vi "Main.vi"() -> ()   [LabVIEW 2018]
uses:
  Source/SG/Typedefs/Waveform Timing Configuration.ctl
  Source/SG/Typedefs/Instrument Configuration.ctl
  <instrlib>/niRFSG/niRFSG.llb/niRFSG Ref Clock Sources.ctl
  <instrlib>/niRFSG/niRFSG.llb/niRFSG Trigger Terminals.ctl
  Source/SG/Typedefs/PAEN Configuration.ctl
  <instrlib>/niRFSG/niRFSG.llb/niRFSG Exported Signal Destinations.ctl
  <instrlib>/niDigital/niDigital.llb/niDigital Burst Pattern (Burst Only).vi
  Source/SG/SG.lvlib
  Source/Digital/Digital.lvlib
panel:
  in  "Configurations":enum32{"Hardware", "Waveform Generation"}(tab)=enum."Waveform Generation"
  in  "RFSG Resource":refnum<k15>="VST2"
  in  "NI Digital Resource":refnum<k15>="PXIe-6570"
  in  "Waveform Timing Configuration":T1={"Duty Cycle (%)"=99.0, "Pre-Burst Time (s)"=1e-06, "Post-Burst Time (s)"=1e-06} {"Post-Burst Time (s)" format="%#_6p"; "Pre-Burst Time (s)" format="%#_6p"; "Duty Cycle (%)" min=1.0 max=100.0 step=1.0 format="%#_2d%%"}
  in  "Waveform File Path":path
  in  "External Attenuation (dB)":dbl
  in  "DUT Average Input Power (dBm)":dbl=-20.0
  in  "Carrier Frequency (Hz)":dbl=1000000000.0 format="%#_6p"
  in  "stop":bool
  out "Status":string
  # "Only supports NI-5840 for generation"
  # "Will use local file if empty"
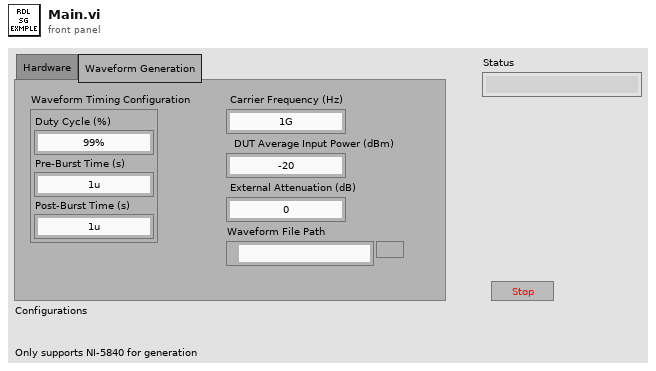
[diagram p1: front panel]
types:
  T1 = typedef "SG.lvlib/Waveform Timing Configuration.ctl" = cluster{"Duty Cycle (%)":dbl, "Pre-Burst Time (s)":dbl, "Post-Burst Time (s)":dbl}
  T2 = typedef "SG.lvlib/Instrument Configuration.ctl" = cluster{"Reference Clock Source":T3, "Carrier Frequency (Hz)":dbl, "DUT Average Input Power (dBm)":dbl, "External Attenuation (dB)":dbl, "Marker 0 Export Terminal":T4, "Share LO  SG->SA":bool}
  T3 = typedef "niRFSG Ref Clock Sources.ctl" = string
  T4 = typedef "niRFSG Trigger Terminals.ctl" = string
  T5 = typedef "SG.lvlib/PAEN Configuration.ctl" = cluster{"PAEN Mode":enum16{"Disabled", "Static", "Dynamic"}, "Command Enable Time (s)":dbl, "Command Disable Time (s)":dbl, "PA Enable Trigger Mode":i32, "PA Enable Trigger Export Terminal":T6}
  T6 = typedef "niRFSG Exported Signal Destinations.ctl" = string
  T7 = cluster{"Generation":cluster{"SG Configuration":T2, "Timing Configuration":T1, "PAEN Configuration":T5}, "Example Folder Path":path}
  T8 = typedef "SG.lvlib/Waveform.ctl" = cluster{"Waveform Name":string, "Waveform":cluster{"x0":dbl, "dx":dbl, "y":csg[]}, "Signal Bandwidth (Hz)":dbl, "PAPR (dB)":dbl, "Burst Length (s)":dbl, "Sample Rate":dbl, "Burst Start Locations":i32[], "Burst Stop Locations":i32[], "Idle Duration Present?":bool}
  T9 = typedef "Digital.lvlib/Project Files.ctl" = cluster{"Pin Map File":path, "Specifications Files":path[], "Pin Levels Files":path[], "Timing Files":path[], "Digital Pattern Files":path[]}
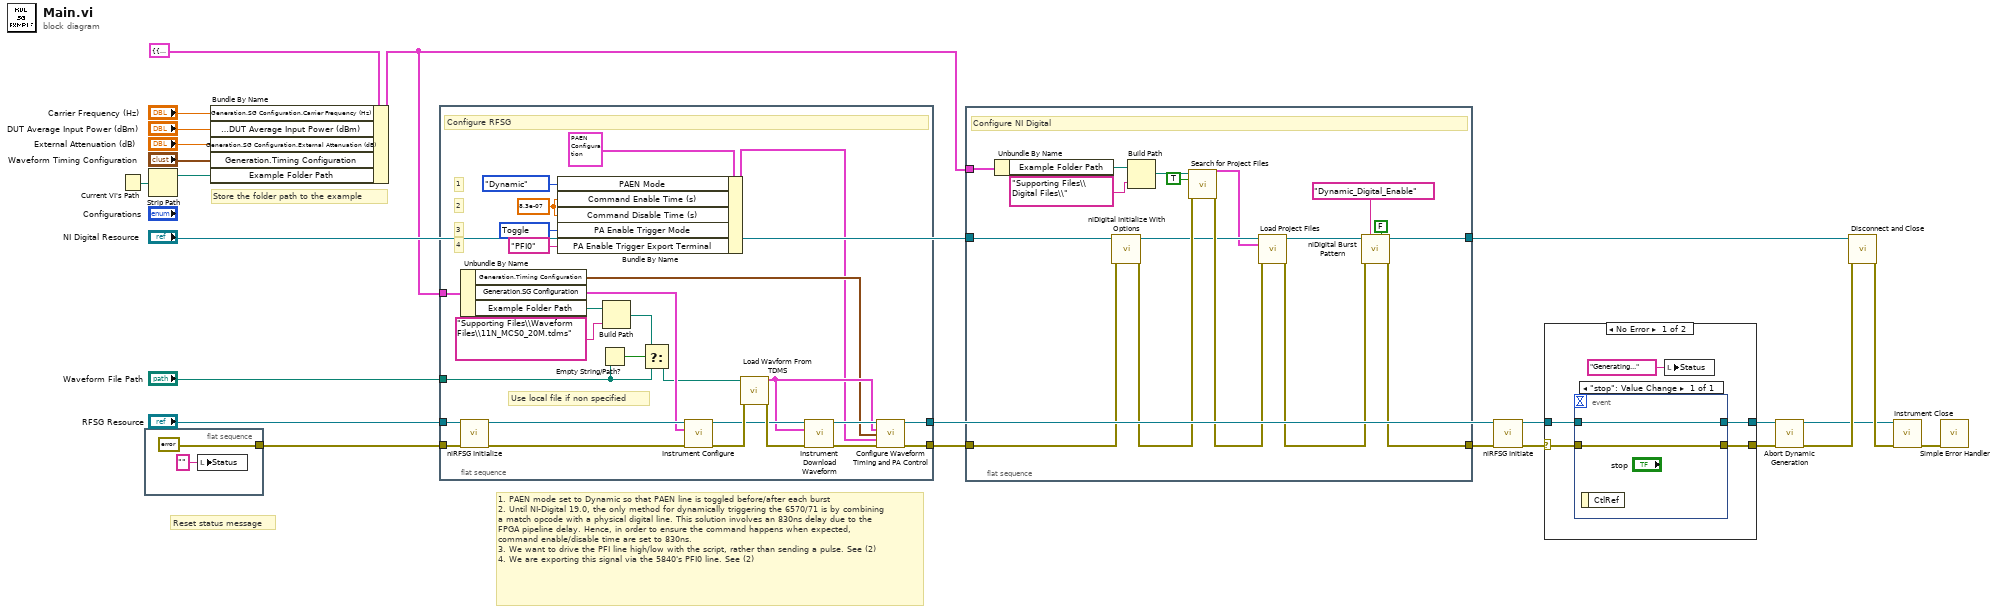
[diagram p0: block diagram]
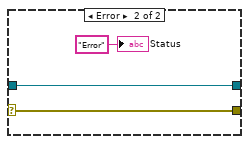
[diagram p2: hidden frame]
diagram:
  # "Reset status message"
  # "1. PAEN mode set to Dynamic so that PAEN line is toggled before/after each burst\n2. Until NI-Digital 19.0, the only method for dynamically triggering the 6570/71 is by combining a match opcode with a physical digital line. This solution involves an 830ns delay due to the FPGA pipeline delay. Hence, in order to ensure the command happens when expected, command enable/disable time are set to 830ns.\n3. We want to drive the PFI line high/low with the script, rather than sending a pulse. See (2)\n4. We are exporting this signal via the 5840's PFI0 line. See (2)"
  # "Store the folder path to the example"
  n1 = Current VI's Path() -> (path=w8:path)
  n2 = flat-sequence {
    tunnel: [errorcluster {"status"=FALSE, "code"=0, "source"=""} ("error constant")] -> w1
    frame #0 {
      n3 = local write "Status"("" ("Status")) -> ()
    }
  }
  n4 = Strip Path(path=w8) -> (stripped path=w6:path)  [unwired: 1 out]
  n5 = Bundle By Name(cluster=T7 {"Generation"={"SG Configuration"={"Reference Clock Source"="OnboardClock", "Carrier Frequency (Hz)"=1000000000.0, "DUT Average Input Power (dBm)"=-20.0, "External Attenuation (dB)"=0.0, "Marker 0 Export Terminal"="PXI_Trig0", "Share LO  SG->SA"=TRUE}, "Timing Configuration"={"Duty Cycle (%)"=50.0, "Pre-Burst Time (s)"=1e-06, "Post-Burst Time (s)"=1e-06}, "PAEN Configuration"={"PAEN Mode"=enum."Dynamic", "Command Enable Time (s)"=0.0, "Command Disable Time (s)"=0.0, "PA Enable Trigger Mode"=23001, "PA Enable Trigger Export Terminal"="PFI0"}}, "Example Folder Path"=path ""}, "Generation.SG Configuration.Carrier Frequency (Hz)"="Carrier Frequency (Hz)", "Generation.SG Configuration.DUT Average Input Power (dBm)"="DUT Average Input Power (dBm)", "Generation.SG Configuration.External Attenuation (dB)"="External Attenuation (dB)", "Generation.Timing Configuration"="Waveform Timing Configuration", "Example Folder Path"=w6) -> (w5:T7)
  n6 = flat-sequence {
    tunnel: [w49] -> w21
    tunnel: [w47] -> w17
    tunnel: "RFSG Resource" -> [w43]
    tunnel: "Waveform File Path" -> [w28]
    tunnel: w5 -> [w42]
    tunnel: w1 -> [w27]
    frame #0 {
      w35 = 23001 items=["Pulse"=23000, "Toggle"=23001] ("PA Enable Trigger Mode")
      w34 = 8.3e-07 ("Command Enable Time (s)")
      # "Use local file if non specified"
      # "4"
      # "3"
      # "2"
      # "1"
      # "Configure RFSG"
      n7 = Unbundle By Name(w42) -> ("Generation.Timing Configuration"=w40:T1, "Generation.SG Configuration"=w41:T2, "Example Folder Path"=w33:path)
      n8 = call <instrlib>:"niRFSG Initialize.vi"("resource name"=w43, "error in"=w27) -> ("instrument handle"=w48:refnum<k15>, "error out"=w53:errorcluster)  [unwired: 12 in]
      n9 = Bundle By Name(cluster=T5 {"PAEN Mode"=enum."Dynamic", "Command Enable Time (s)"=8.3e-07, "Command Disable Time (s)"=8.3e-07, "PA Enable Trigger Mode"=23001, "PA Enable Trigger Export Terminal"="PXI_Trig1"} ("PAEN Configuration"), "PAEN Mode"=enum16{"Disabled", "Static", "Dynamic"}."Dynamic", "Command Enable Time (s)"=w34, "Command Disable Time (s)"=w34, "PA Enable Trigger Mode"=w35, "PA Enable Trigger Export Terminal"=T6 "PFI0") -> (w38:T5)
      n10 = Empty String/Path?(string/path=w28) -> (empty?=w31:bool)
      n11 = Build Path(base path=w33, name or relative path="Supporting Files\\Waveform Files\\11N_MCS0_20M.tdms") -> (appended path=w30:path)
      n12 = Select(t=w30, s=w31, f=w28) -> (s? t:f=w29:path)
      n13 = call "Instrument Configure.vi"("RFSG Session In"=w48, "SG Configuration"=w41, "error in (no error)"=w53) -> ("RFSG Session Out"=w46:refnum<k15>, "error out"=w51:errorcluster)  [unwired: 11 in]
      n14 = call "Load Wavform From TDMS.vi"("TDMS File Path"=w29, "error in (no error)"=w51) -> ("Waveform"=w44:T8, "error out"=w50:errorcluster)  [unwired: 12 in]
      n15 = call "Instrument Download Waveform.vi"("RFSG handle"=w46, "Waveform In"=w44, "error in (no error)"=w50) -> ("RFSG handle out"=w45:refnum<k15>, "error out"=w52:errorcluster)  [unwired: 11 in]
      n16 = call "Configure Waveform Timing and PA Control.vi"("RFSG handle"=w45, "Waveform"=w44, "Waveform Timing Configuration"=w40, "PAEN Configuration"=w38, "error in"=w52) -> ("RFSG handle out"=w47:refnum<k15>, "error out"=w49:errorcluster)  [unwired: 8 in, 1 out]
    }
  }
  n17 = flat-sequence {
    tunnel: w21 -> [w70]
    tunnel: [w56] -> w20
    tunnel: "NI Digital Resource" -> [w67]
    tunnel: [w58] -> w9
    tunnel: w5 -> [w60]
    frame #0 {
      # "Configure NI Digital"
      n18 = Unbundle By Name(w60) -> ("Example Folder Path"=w59:path)
      n19 = call <instrlib>:"niDigital Initialize With Options.vi"("resource name"=w67, "error in"=w70) -> ("instrument handle"=w65:refnum<k15>, "error out"=w69:errorcluster)  [unwired: 12 in]
      n20 = Build Path(base path=w59, name or relative path="Supporting Files\\Digital Files\\") -> (appended path=w61:path)
      n21 = call "Search for Project Files.vi"("Search Directory"=w61, "Recursive Search? (F)"=TRUE, "error in (no error)"=w69) -> ("Project Files"=w64:T9, "error out"=w68:errorcluster)  [unwired: 11 in]
      n22 = call "Load Project Files.vi"("NI Digital in"=w65, "Project Files"=w64, "error in (no error)"=w68) -> ("NI Digital out"=w63:refnum<k15>, "error out"=w57:errorcluster)  [unwired: 11 in]
      n23 = call-poly <instrlib>:"niDigital Burst Pattern.vi"("instrument handle"=w63, "start label"="Dynamic_Digital_Enable", "wait until done? (T)"=FALSE, "error in"=w57) -> ("instrument handle out"=w58:refnum<k15>, "error out"=w56:errorcluster)  [unwired: 10 in]
    }
  }
  n24 = call <instrlib>:"niRFSG Initiate.vi"("instrument handle"=w17, "error in"=w20) -> ("instrument handle out"=w15:refnum<k15>, "error out"=w22:errorcluster)  [unwired: 12 in]
  n25 = case shown="No Error" w22 {
    selector: w22 -> [w74 w80]
    tunnel: w15 -> [w73 w79]
    tunnel: [w72 w79] -> w14
    tunnel: [w75 w80] -> w24
    frame No Error {
      n26 = event shown="[0] \"stop\": Value Change" {
        selector: _ -> [_]
        dyn-events: _ -> [_]
        timeout: _ -> [_]
        tunnel: w74 -> [w77]
        tunnel: w73 -> [w76]
        tunnel: [w76] -> w72
        tunnel: [w77] -> w75
        event "stop": Value Change {
          n27 = event-data() -> ()  [unwired: 1 in, 1 out]
        }
      }
      n28 = local write "Status"("Generating..." ("Status")) -> ()
    }
    frame Error {
      "Status" <- "Error" ("Status")
    }
  }
  n29 = call "Abort Dynamic Generation.vi"("RFSG handle"=w14, "error in (no error)"=w24) -> ("RFSG handle out"=w16:refnum<k15>, "error out"=w19:errorcluster)  [unwired: 12 in]
  n30 = call "Disconnect and Close.vi"("NI Digital in"=w9, "error in (no error)"=w19) -> ("error out"=w18:errorcluster)  [unwired: 13 in]
  n31 = call "Instrument Close.vi"("RFSG Handle"=w16, "error in (no error)"=w18) -> ("error out"=w23:errorcluster)  [unwired: 13 in]
  n32 = call <vilib>:"Simple Error Handler.vi"("error in (no error)"=w23) -> ()  [unwired: 4 in, 5 out]
